vi "test_libssh2_sftp_readdir_attr.vi"() -> ()   [LabVIEW 2017, in "integration_tests.lvlib"]
uses:
  integration_tests.lvlib
  libssh2/libssh2_sftp_open_ex.vi
  libssh2/libssh2_sftp_readdir_ex.vi
  libssh2/libssh2_sftp_close_handle.vi
  support/support.lvlib
  libssh2/libssh2.lvlib
  <vilib>/PNR/Transparent Assertions/Transparent Assertions/Transparent Assertions.lvlib
panel:
  out "error out":errorcluster
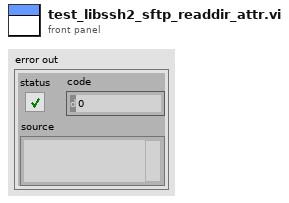
[diagram p1: front panel]
types:
  T1 = typedef "libssh2.lvlib/Session Refnum.ctl" = refnum<k1>
  T2 = typedef "libssh2.lvlib/SFTP Refnum.ctl" = refnum<k1>
  T3 = typedef "libssh2.lvlib/SFTP Handle Refnum.ctl" = refnum<k1>
  T4 = typedef "libssh2.lvlib/libssh2_sftp_attributes.ctl" = cluster{"flags":u32, "filesize":u64, "uid":u32, "gid":u32, "permissions":u32, "atime":u32, "mtime":u32}
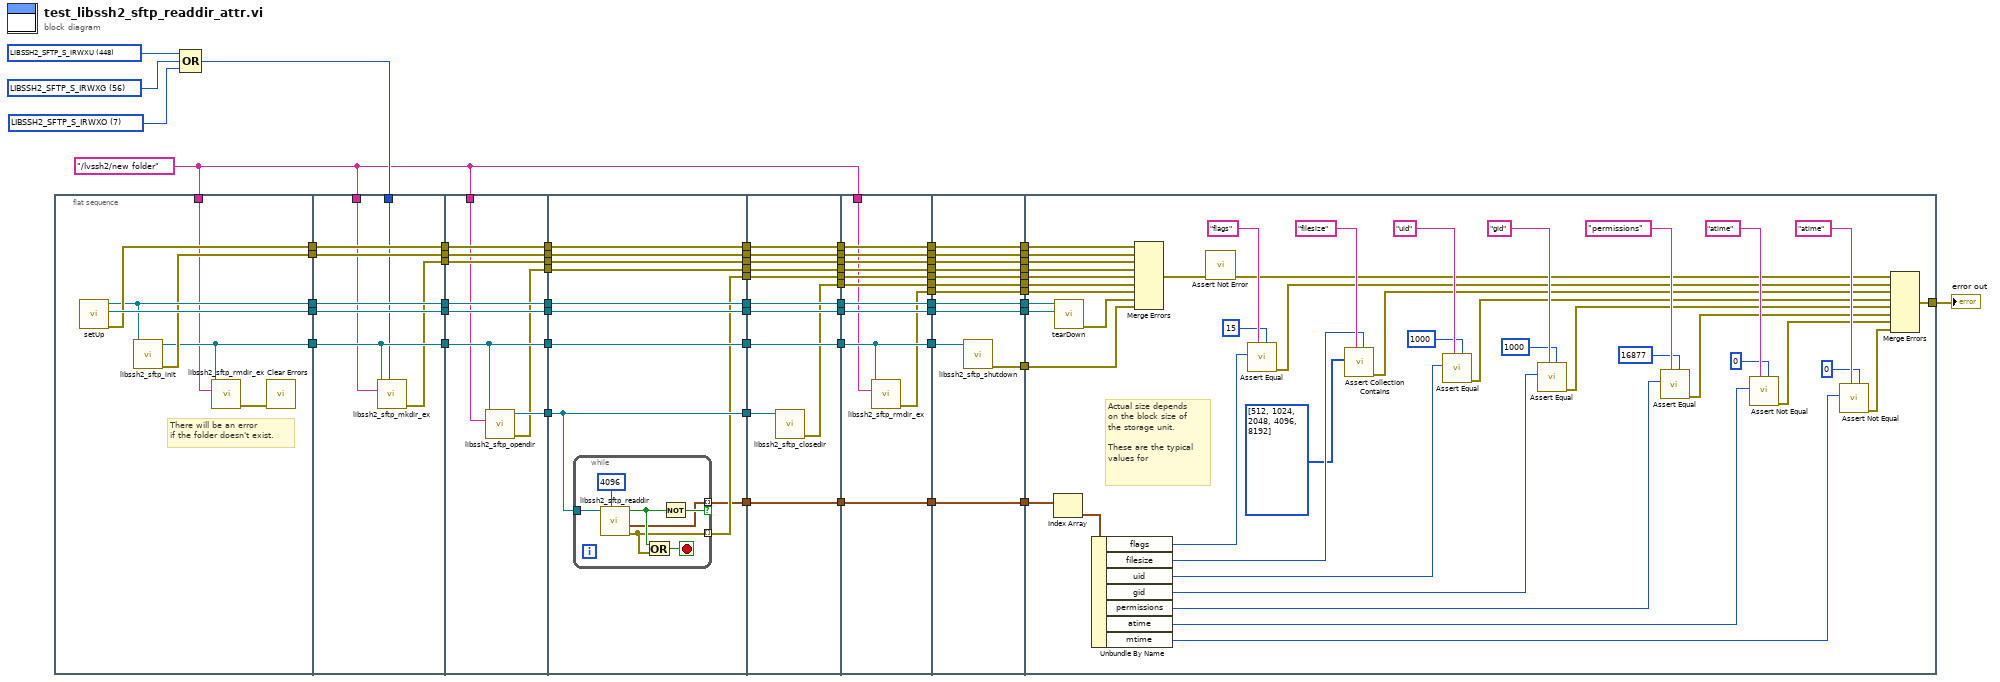
[diagram p0: block diagram]
diagram:
  w3 = "/lvssh2/new folder" ("filename")
  w59 = 7 items=["LIBSSH2_SFTP_S_IRWXU"=448, "LIBSSH2_SFTP_S_IRUSR"=256, "LIBSSH2_SFTP_S_IWUSR"=128, "LIBSSH2_SFTP_S_IXUSR"=64, "LIBSSH2_SFTP_S_IRWXG"=56, "LIBSSH2_SFTP_S_IRGRP"=32, "LIBSSH2_SFTP_S_IWGRP"=16, "LIBSSH2_SFTP_S_IXGRP"=8, "LIBSSH2_SFTP_S_IRWXO"=7, "LIBSSH2_SFTP_S_IROTH"=4, "LIBSSH2_SFTP_S_IWOTH"=2, "LIBSSH2_SFTP_S_IXOTH"=1] ("mode")
  w60 = 56 items=["LIBSSH2_SFTP_S_IRWXU"=448, "LIBSSH2_SFTP_S_IRUSR"=256, "LIBSSH2_SFTP_S_IWUSR"=128, "LIBSSH2_SFTP_S_IXUSR"=64, "LIBSSH2_SFTP_S_IRWXG"=56, "LIBSSH2_SFTP_S_IRGRP"=32, "LIBSSH2_SFTP_S_IWGRP"=16, "LIBSSH2_SFTP_S_IXGRP"=8, "LIBSSH2_SFTP_S_IRWXO"=7, "LIBSSH2_SFTP_S_IROTH"=4, "LIBSSH2_SFTP_S_IWOTH"=2, "LIBSSH2_SFTP_S_IXOTH"=1] ("mode")
  w61 = 448 items=["LIBSSH2_SFTP_S_IRWXU"=448, "LIBSSH2_SFTP_S_IRUSR"=256, "LIBSSH2_SFTP_S_IWUSR"=128, "LIBSSH2_SFTP_S_IXUSR"=64, "LIBSSH2_SFTP_S_IRWXG"=56, "LIBSSH2_SFTP_S_IRGRP"=32, "LIBSSH2_SFTP_S_IWGRP"=16, "LIBSSH2_SFTP_S_IXGRP"=8, "LIBSSH2_SFTP_S_IRWXO"=7, "LIBSSH2_SFTP_S_IROTH"=4, "LIBSSH2_SFTP_S_IWOTH"=2, "LIBSSH2_SFTP_S_IXOTH"=1] ("mode")
  n1 = flat-sequence {
    tunnel: [w72] -> w67
    tunnel: [w74] -> w66
    tunnel: [w73] -> w65
    tunnel: [w71] -> w63
    tunnel: [w70] -> w62
    tunnel: w3 -> [w69]
    tunnel: w67 -> [w82]
    tunnel: w66 -> [w81]
    tunnel: [w82] -> w50
    tunnel: [w81] -> w49
    tunnel: [w78] -> w48
    tunnel: [w80] -> w47
    tunnel: w65 -> [w80]
    tunnel: w63 -> [w79]
    tunnel: [w79] -> w46
    tunnel: w62 -> [w78]
    tunnel: w58 -> [w77]
    tunnel: w3 -> [w76]
    tunnel: [w75] -> w45
    tunnel: w50 -> [w91]
    tunnel: [w91] -> w42
    tunnel: w49 -> [w90]
    tunnel: [w90] -> w40
    tunnel: w48 -> [w86]
    tunnel: [w86] -> w38
    tunnel: w47 -> [w89]
    tunnel: [w89] -> w36
    tunnel: w46 -> [w88]
    tunnel: [w88] -> w34
    tunnel: w45 -> [w87]
    tunnel: [w87] -> w32
    tunnel: w3 -> [w85]
    tunnel: [w84] -> w30
    tunnel: [w83] -> w28
    tunnel: w42 -> [w101]
    tunnel: [w101] -> w41
    tunnel: w40 -> [w100]
    tunnel: [w100] -> w39
    tunnel: w38 -> [w99]
    tunnel: [w99] -> w37
    tunnel: w36 -> [w98]
    tunnel: [w98] -> w35
    tunnel: w34 -> [w97]
    tunnel: [w97] -> w33
    tunnel: w32 -> [w96]
    tunnel: [w96] -> w31
    tunnel: w30 -> [w94]
    tunnel: [w94] -> w29
    tunnel: w28 -> [w95]
    tunnel: [w95] -> w27
    tunnel: [w93] -> w26
    tunnel: [w92] -> w24
    tunnel: w41 -> [w119]
    tunnel: [w119] -> w23
    tunnel: w39 -> [w118]
    tunnel: [w118] -> w21
    tunnel: w37 -> [w117]
    tunnel: [w117] -> w19
    tunnel: w35 -> [w116]
    tunnel: [w116] -> w17
    tunnel: w33 -> [w115]
    tunnel: [w115] -> w15
    tunnel: w31 -> [w114]
    tunnel: [w114] -> w13
    tunnel: w29 -> [w113]
    tunnel: [w109] -> w11
    tunnel: w27 -> [w112]
    tunnel: [w112] -> w9
    tunnel: [w111] -> w7
    tunnel: w26 -> [w110]
    tunnel: [w110] -> w5
    tunnel: w24 -> [w109]
    tunnel: w23 -> [w131]
    tunnel: [w131] -> w22
    tunnel: w21 -> [w130]
    tunnel: [w130] -> w20
    tunnel: w19 -> [w122]
    tunnel: [w122] -> w18
    tunnel: w17 -> [w129]
    tunnel: [w129] -> w16
    tunnel: w15 -> [w128]
    tunnel: [w128] -> w14
    tunnel: w13 -> [w127]
    tunnel: [w127] -> w12
    tunnel: w11 -> [w126]
    tunnel: [w126] -> w10
    tunnel: w9 -> [w125]
    tunnel: [w125] -> w8
    tunnel: w7 -> [w124]
    tunnel: [w124] -> w6
    tunnel: w5 -> [w123]
    tunnel: [w123] -> w4
    tunnel: w3 -> [w121]
    tunnel: [w120] -> w2
    tunnel: w22 -> [w143]
    tunnel: [w143] -> w57
    tunnel: w20 -> [w142]
    tunnel: [w142] -> w56
    tunnel: w18 -> [w139]
    tunnel: [w136] -> w55
    tunnel: w16 -> [w141]
    tunnel: [w141] -> w54
    tunnel: w14 -> [w140]
    tunnel: [w140] -> w53
    tunnel: [w138] -> w52
    tunnel: w12 -> [w137]
    tunnel: [w137] -> w51
    tunnel: [w135] -> w44
    tunnel: w10 -> [w136]
    tunnel: w8 -> [w135]
    tunnel: w6 -> [w134]
    tunnel: [w134] -> w43
    tunnel: w4 -> [w133]
    tunnel: [w133] -> w25
    tunnel: w2 -> [w132]
    tunnel: [w132] -> w1
    tunnel: w57 -> [w187]
    tunnel: w56 -> [w186]
    tunnel: w55 -> [w176]
    tunnel: w54 -> [w185]
    tunnel: [w146] -> w64
    tunnel: w53 -> [w183]
    tunnel: w52 -> [w182]
    tunnel: w51 -> [w181]
    tunnel: w44 -> [w180]
    tunnel: w43 -> [w179]
    tunnel: w25 -> [w178]
    tunnel: w1 -> [w177]
    frame #0 {
      # "There will be an error\nif the folder doesn't exist."
      n2 = call "setUp.vi"() -> ("error out"=w73:errorcluster, "connection ID"=w74:refnum<k5>, "session"=w72:T1)  [unwired: 9 in]
      n3 = call "libssh2_sftp_init.vi"("session"=w72) -> ("error out"=w71:errorcluster, "sftp"=w70:T2)  [unwired: 9 in]
      n4 = call "libssh2_sftp_rmdir_ex.vi"("path"=w69, "sftp"=w70) -> ("error out"=w68:errorcluster)  [unwired: 9 in]
      n5 = call <vilib>:"Clear Errors.vi"("error in (no error)"=w68) -> ()  [unwired: 5 in, 2 out]
    }
    frame #1 {
      n6 = call "libssh2_sftp_mkdir_ex.vi"("mode"=w77, "path"=w76, "sftp"=w78) -> ("error out"=w75:errorcluster)  [unwired: 8 in]
    }
    frame #2 {
      n7 = call "libssh2_sftp_opendir.vi"("path"=w85, "sftp"=w86) -> ("error out"=w83:errorcluster, "sftp handle"=w84:T3)  [unwired: 8 in]
    }
    frame #3 {
      n8 = while {
        tunnel: w94 -> [w108]
        tunnel: [w103] -> w93 mode=indexing
        tunnel: [w102] -> w92 mode=indexing if=w106
        stop <- w105 stop-if-true
        n9 = call "libssh2_sftp_readdir.vi"("buffer maxlen"=4096, "sftp handle"=w108) -> ("error out"=w103:errorcluster, "attrs"=w102:T4, "no more files"=w104:bool)  [unwired: 6 in, 1 out]
        n10 = Or(x=w104, y=w103) -> (x .or. y?=w105:bool)
        n11 = Not(x=w104) -> (.not. x?=w106:bool)
      }
    }
    frame #4 {
      n12 = call "libssh2_sftp_closedir.vi"("sftp handle"=w113) -> ("error out"=w111:errorcluster)  [unwired: 10 in]
    }
    frame #5 {
      n13 = call "libssh2_sftp_rmdir_ex.vi"("path"=w121, "sftp"=w122) -> ("error out"=w120:errorcluster)  [unwired: 9 in]
    }
    frame #6 {
      n14 = call "libssh2_sftp_shutdown.vi"("sftp"=w139) -> ("error out"=w138:errorcluster)  [unwired: 10 in]
    }
    frame #7 {
      # "Actual size depends\non the block size of\nthe storage unit.\n\nThese are the typical\nvalues for"
      n15 = Index Array(array=w176) -> (element=w175:T4)  [unwired: 1 in]
      n16 = call "tearDown.vi"("connection ID"=w186, "session"=w187) -> ("error out"=w184:errorcluster)  [unwired: 9 in]
      n17 = Unbundle By Name(w175) -> ("flags"=w166:u32, "filesize"=w145:u64, "uid"=w165:u32, "gid"=w163:u32, "permissions"=w161:u32, "atime"=w159:u32, "mtime"=w157:u32)
      n18 = Merge Errors(w185, w183, w181, w180, w178, w179, w177, w184, w182) -> (w155:errorcluster)
      n19 = call <vilib>:"Assert Not Error.vi"("error in (no error)"=w155) -> ("error out"=w154:errorcluster)  [unwired: 10 in]
      n20 = call <vilib>:"Assert Equal.vi"("Expected"=u32 15, "Message (\"\")"="flags" ("Label"), "Actual"=w166) -> ("error out"=w153:errorcluster)  [unwired: 8 in]
      n21 = call <vilib>:"Assert Collection Contains.vi"("Expected"=w145, "Message (\"\")"="filesize" ("Label"), "Collection"=u64[] [512, 1024, 2048, 4096, 8192]) -> ("error out"=w152:errorcluster)  [unwired: 8 in]
      n22 = call <vilib>:"Assert Equal.vi"("Expected"=u32 1000, "Message (\"\")"="uid" ("Label"), "Actual"=w165) -> ("error out"=w151:errorcluster)  [unwired: 8 in]
      n23 = call <vilib>:"Assert Equal.vi"("Expected"=u32 1000, "Message (\"\")"="gid" ("Label"), "Actual"=w163) -> ("error out"=w150:errorcluster)  [unwired: 8 in]
      n24 = call <vilib>:"Assert Equal.vi"("Expected"=u32 16877, "Message (\"\")"="permissions" ("Label"), "Actual"=w161) -> ("error out"=w149:errorcluster)  [unwired: 8 in]
      n25 = call <vilib>:"Assert Not Equal.vi"("Expected"=u32 0, "Message (\"\")"="atime" ("Label"), "Actual"=w159) -> ("error out"=w148:errorcluster)  [unwired: 8 in]
      n26 = call <vilib>:"Assert Not Equal.vi"("Expected"=u32 0, "Message (\"\")"="atime" ("Label"), "Actual"=w157) -> ("error out"=w147:errorcluster)  [unwired: 8 in]
      n27 = Merge Errors(w154, w153, w152, w151, w150, w149, w148, w147) -> (w146:errorcluster)
    }
  }
  n28 = Compound Arithmetic op=OR(w61, w60, w59) -> (w58:i32)
  "error out" <- w64
